vi "dataHandler_sub.vi"(0 "Instance":i32, 1 "Latest?":bool) -> (7 "instance out":i32, 8 "dataToRead?":bool)   [LabVIEW 2023]
uses:
  LVLib/SADI_FW3.lvlib
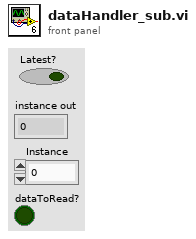
[diagram p1: front panel]
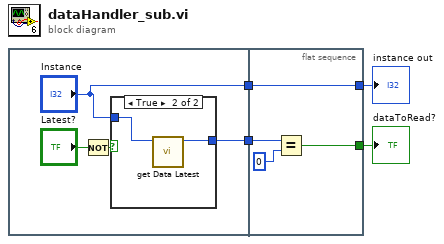
[diagram p0: block diagram]
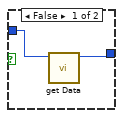
[diagram p2: hidden frame]
diagram:
  n1 = flat-sequence {
    tunnel: [w6] -> w4
    tunnel: ["Instance"] -> w3
    tunnel: w4 -> [w16]
    tunnel: [w14] -> w1
    tunnel: [w13] -> w2
    tunnel: w3 -> [w13]
    frame #0 {
      n2 = Not(x="Latest?") -> (.not. x?=w8:bool)
      n3 = case shown="True" w8 {
        tunnel: [w10 w12] -> w6
        tunnel: "Instance" -> [w9 w11]
        frame False {
          n4 = call "get Data.vi"("instance"=w9) -> ("function return"=w10:u32)  [unwired: 10 in]
        }
        frame True {
          n5 = call "get Data Latest.vi"("instance"=w11) -> ("function return"=w12:u32)  [unwired: 10 in]
        }
      }
    }
    frame #1 {
      n6 = Equal?(x=w16, y=u32 0) -> (x = y?=w14:bool)
    }
  }
  "instance out" <- w2
  "dataToRead?" <- w1
